vi "Delete_Row_Data.vi"(6 "Country":string, 11 "Raw Data Array (String)":string[][](array[string])) -> (3 "array w/ subset deleted":string[][](array[string]))   [LabVIEW 2015]
doc: "This VI deletes data from duplicate countries from the 2D-array of strings"
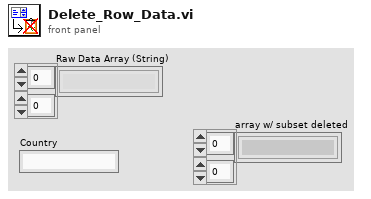
[diagram p1: front panel]
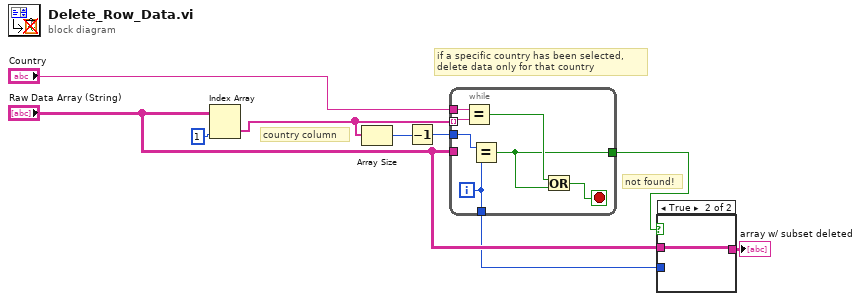
[diagram p0: block diagram]
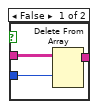
[diagram p2: hidden frame]
diagram:
  # "not found!"
  # "if a specific country has been selected, \ndelete data only for that country"
  # "country column"
  n1 = Index Array(array="Raw Data Array (String)", index (col)=1 ("index (row)")) -> (element=w7:string[])  [unwired: 1 in]
  n2 = Array Size(array=w7) -> (size(s)=w6:i32)
  n3 = Decrement(x=w6) -> (x-1=w5:i32)
  n4 = while {
    tunnel: w7 -> [w15] mode=indexing
    tunnel: "Country" -> [w16]
    tunnel: "Raw Data Array (String)" -> [_]
    tunnel: w5 -> [w12]
    tunnel: [w11] -> w1
    tunnel: [w10] -> w3
    i -> [w10]
    stop <- w14 stop-if-true
    n5 = Equal?(x=w16, y=w15) -> (x = y?=w13:bool)
    n6 = Equal?(x=w12, y=w10) -> (x = y?=w11:bool)
    n7 = Or(x=w13, y=w11) -> (x .or. y?=w14:bool)
  }
  n8 = case shown="True" w1 {
    tunnel: "Raw Data Array (String)" -> [w19 w20]
    tunnel: w3 -> [w18 _]
    tunnel: [w17 w20] -> w2
    frame False {
      n9 = Delete From Array(array=w19, index (row)=w18) -> (array with subset deleted=w17:string[][])  [unwired: 2 in, 1 out]
    }
    frame True {
    }
  }
  "array w/ subset deleted" <- w2
